vi "Keyence.File.Write.vi"(8 "error in":errorcluster, 11 "segtings path":path) -> (0 "error out":errorcluster)   [LabVIEW 2016]
uses:
  tools/Tma.lib/nlconfig.llb/fp2ini mode.ctl
  Keyence.Global.vi
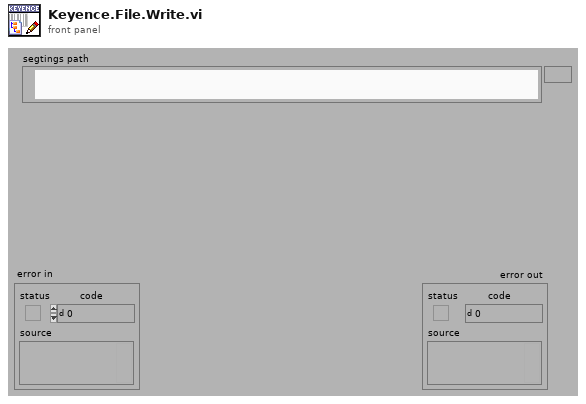
[diagram p1: front panel]
types:
  T1 = typedef "fp2ini mode.ctl" = enum16{"Read Controls", "Write Controls", "Write Indicators", "Read Indicators", "Write all", "Read all"}
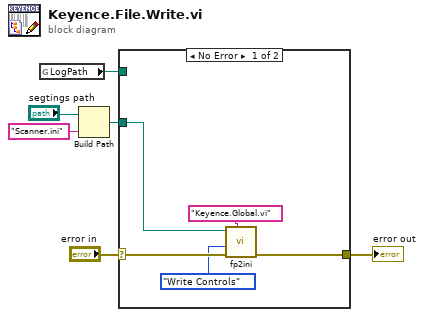
[diagram p0: block diagram]
diagram:
  n1 = global read "Keyence.Global.vi" "LogPath"() -> (w1:path)
  n2 = Build Path(base path="segtings path", name or relative path="Scanner.ini") -> (appended path=w3:path)
  n3 = case shown="No Error" "error in" {
    selector: "error in" -> [w11 w12]
    tunnel: [w8 w12] -> w6
    tunnel: w3 -> [w10 _]
    tunnel: w1 -> [_ _]
    frame No Error {
      n4 = call "fp2ini.vi"("vi-name (caller if empty)"="Keyence.Global.vi", "error in"=w11, "mode"=fp2ini_mode."Write Controls", "ini-file path"=w10) -> ("error out"=w8:errorcluster)  [unwired: 3 in, 4 out]
    }
    frame Error {
    }
  }
  "error out" <- w6
